vi "Test Create Start Stop Destroy.vi"() -> ()   [LabVIEW 2019, in "instrument.PPMS.lvclass"]
uses:
  instrument.PPMS.lvclass
  PPMS/PPMS.lvlib
  <vilib>/JKI/JKI SMO/SMO/SMO.lvclass
  C:/Program Files (x86)/National Instruments/LabVIEW 2019/user.lib/LevyLab/Instrument Framework/Instrument Types/Cryostat/Instrument.Cryostat.lvclass
  C:/Program Files (x86)/National Instruments/LabVIEW 2019/user.lib/LevyLab/Instrument Framework/Instrument/Instrument.lvclass
  C:/Program Files (x86)/National Instruments/LabVIEW 2019/vi.lib/JKI/JKI SMO/SMO/SMO.lvclass
  <userlib>/LevyLab/Instrument Framework/Instrument/Instrument.lvclass
  PPMS/Select PPMS--Enum.ctl
panel:
  in  "Select PPMS":T1=enum."Simulate PPMS"
  in  "Debug Mode?":bool
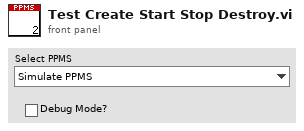
[diagram p1: front panel]
types:
  T1 = typedef "PPMS.lvlib/Select PPMS--Enum.ctl" = enum16{"PPMS1", "PPMS2", "PPMS3", "OptiCool", "Simulate PPMS", "Simulate OptiCool"}
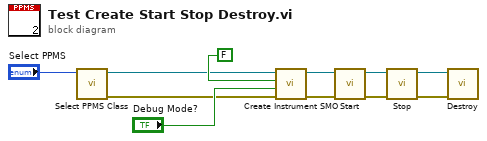
[diagram p0: block diagram]
diagram:
  n1 = call "Select PPMS Class.vi"("Select PPMS"="Select PPMS") -> ("error out"=w8:errorcluster, "instrument.PPMS out"=w9:refnum<class "instrument.PPMS.lvclass">)  [unwired: 9 in]
  n2 = call <userlib>:"Create Instrument SMO.vi"("error in (no error)"=w8, "Debug Mode? [F]"="Debug Mode?", "Configuration Window? [T]"=FALSE, "Instrument in"=w9) -> ("error out"=w6:errorcluster, "Instrument out"=w5:refnum<class "instrument.PPMS.lvclass">)  [unwired: 6 in]
  n3 = call <vilib>:"Start.vi"("error in (no error)"=w6, "SMO"=w5) -> ("error out"=w4:errorcluster, "SMO out"=w3:refnum<class "instrument.PPMS.lvclass">)  [unwired: 8 in]
  n4 = call <vilib>:"Stop.vi"("error in (no error)"=w4, "SMO"=w3) -> ("error out"=w1:errorcluster, "SMO out"=w2:refnum<class "instrument.PPMS.lvclass">)  [unwired: 8 in]
  n5 = call <vilib>:"Destroy.vi"("error in (no error)"=w1, "SMO"=w2) -> ()  [unwired: 9 in, 1 out]
